vi "CDEx Effect of Controller Type.vi"() -> ()   [LabVIEW 2020]
doc: "This example demonstrate how to calculate the steady-state error for a model with zero, one, or two integrators. This example also demonstrates how to create and simulate a ramp input signal."
uses:
  <vilib>/addons/Control Design/_Model Construction/Data Typedefs.llb/CD Time Info.ctl
  <vilib>/Analysis/1siggen.llb/Ramp Pattern by Samples.vi
  <vilib>/addons/Control Design/_Model Construction/Model Creation.llb/Model Creation SubVI/cd_Create Transfer Function Model.vi
  <vilib>/addons/Control Design/_Utility/Model Viewer.llb/Model Viewer SubVI/cd_Draw Transfer Function Equation (TF).vi
  <vilib>/addons/Control Design/_Model Interconnection/Model Interconnection.llb/Model Interconnection SubVI/cd_Series (TF and TF).vi
  <vilib>/addons/Control Design/_Dynamic Analysis/Dynamic Analysis.llb/Dynamic Analysis subVI/cd_DC Gain (Transfer Function).vi
  <vilib>/addons/Control Design/_Model Interconnection/Model Interconnection.llb/Model Interconnection SubVI/cd_Feedback (TF and TF).vi
  <vilib>/addons/Control Design/_Time Response Analysis/Time Response.llb/Time Response subVI/cd_Linear Simulation (Transfer Function).vi
  <vilib>/addons/Control Design/_Utility/Plots.llb/CD Get IO Time Data.vi
  <vilib>/addons/Control Design/_Time Response Analysis/Time Response.llb/Time Response subVI/cd_Step Response (Transfer Function).vi
  <vilib>/addons/Control Design/_Model Construction/NI_LinSys_Data Typedefs.lvlib
  <vilib>/addons/Control Design/_Dynamic Analysis/NI_CD_Dynamic Analysis.lvlib
  <vilib>/addons/Control Design/_Model Construction/NI_LinSys_Model Creation.lvlib
  <vilib>/addons/Control Design/_Model Interconnection/NI_CD_Model Interconnection.lvlib
  <vilib>/addons/Control Design/_Utility/NI_CD_Model Viewer.lvlib
  <vilib>/addons/Control Design/_Time Response Analysis/NI_CD_Time Response.lvlib
  <vilib>/Analysis/NI_AALBase.lvlib
panel:
  out "Acceleration Error Constant":dbl format="%#.6f"
  out "Steady-state Acceleration Error":dbl=inf format="%#.6f"
  out "Steady-state Velocity Constant (Kv)":dbl=0.27922588002276405 format="%#.6f"
  out "Steady-state Tracking Constant (Kp)":dbl=inf format="%#.6f"
  out "Steady-state Velocity Error":dbl=3.5813299251433084 format="%#.6f"
  out "Steady-state Tracking Error":dbl format="%#.6f"
  in  "Stop":bool
  out "Controller":picture
  in  "Controller Gain":dbl(slide)=0.8376776400682923 scale=0.0001..100.0
  in  "Controller Type":u16(ring)=1 items=["Type 0 - No integrators", "Type 1 - one integrator", "Type 2 - two integrators"]
  out "Plant":picture
  out "Ramp Response":cluster{"time":dbl[], dbl[]}[](graph)
  out "Step Response":cluster{"time":dbl[], dbl[]}[](graph)
  # "Overview: This example demonstrate how to calculate the steady-state error for a model with zero, one, or two integrators.  This example also demonstrates how to create and simulate a ramp input signal.\nInstructions:\n1. Run the VI.\n2. Change the type of Controller and the Controller Gain and verify how this would affect the step and the ramp response. Also, notice that increasing the number of integrators in the plant, it will remove the steady-state error for step or a ramp input signal (u)"
  # "u"
  # "y"
  # "+"
  # "-"
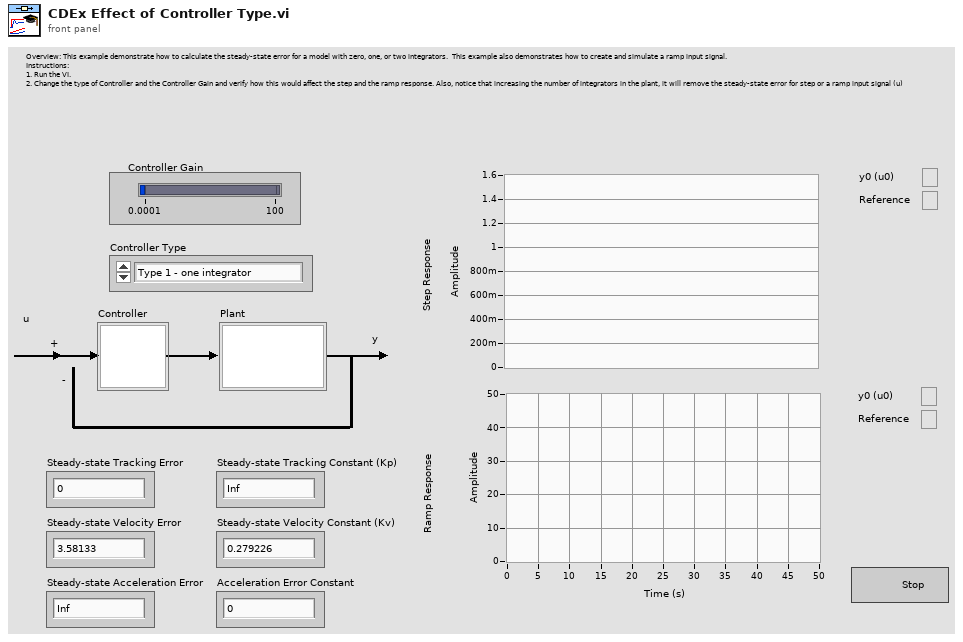
[diagram p1: front panel]
types:
  T1 = typedef "NI_LinSys_Data Typedefs.lvlib/CD Time Info.ctl" = cluster{"t0":dbl, "dt":dbl, "tf":dbl}
  T2 = typedef "NI_LinSys_Model Typedefs.lvlib/CD Transfer Function Model (MIMO).ctl" = cluster{"properties":T3, "transfer function(s)":T4[][]}
  T3 = typedef "NI_LinSys_Model Typedefs.lvlib/CD General Elements.ctl" = cluster{"Model name":string, "Input names":string[], "Output names":string[], "Input Delays":dbl[], "Output Delays":dbl[], "Sampling Time":dbl, "Notes":string}
  T4 = typedef "NI_LinSys_Model Typedefs.lvlib/CD Transfer Function Model (SISO).ctl" = cluster{"Numerator":dbl[], "Denominator":dbl[], "delay":dbl}
  T5 = typedef "NI_LinSys_Data Typedefs.lvlib/CD MIMO Time Response Data.ctl" = cluster{"Time":dbl[], "Outputs Data":dbl[][][], "States Data":dbl[][][], "plot type":T6}
  T6 = typedef "NI_LinSys_Data Typedefs.lvlib/CD Plot Types Enum.ctl" = enum16{"bode-magnitude", "bode-phase", "nichols", "nyquist", "singular values", "step", "impulse", "initial", "simulation", "nyquist with separation"}
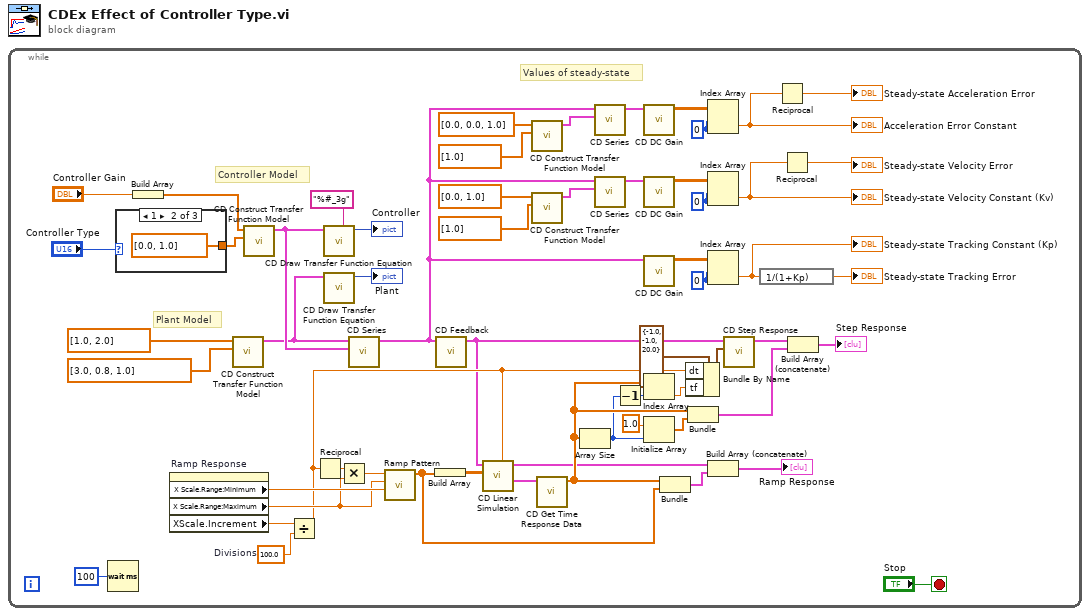
[diagram p0: block diagram]
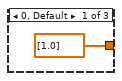
[diagram p2: hidden frame]
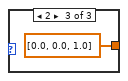
[diagram p3: hidden frame]
diagram:
  n1 = while {
    stop <- "Stop" stop-if-true
    w8 = 0 ("disabled index (col)")
    w20 = 0 ("disabled index (col)")
    w23 = 0 ("disabled index (col)")
    w28 = 100.0  # Divisions
    # "Controller Model"
    # "Plant Model"
    # "Values of steady-state"
    n2 = Wait (ms)(milliseconds to wait=u32 100) -> ()  [unwired: 1 out]
    n3 = case shown="1" "Controller Type" {
      tunnel: [dbl[] [1.0] ("Denominator") dbl[] [0.0, 1.0] ("Denominator") dbl[] [0.0, 0.0, 1.0] ("Denominator")] -> w45
      frame 0, Default {
      }
      frame 1 {
      }
      frame 2 {
      }
    }
    n4 = Build Array("Controller Gain") -> (w39:dbl[])
    n5 = property on="Ramp Response" class="XYGraph (strict)"() -> ("X Scale.Range:Minimum"=w56:dbl, "X Scale.Range:Maximum"=w55:dbl, "XScale.Increment"=w27:dbl)  [unwired: 2 in, 2 out]
    n6 = call-poly <vilib>:"CD Construct Transfer Function Model.vi"("Denominator"=dbl[] [3.0, 0.8, 1.0], "Numerator"=dbl[] [1.0, 2.0]) -> ("Transfer Function Model"=w36:T2)  [unwired: 8 in, 1 out]
    n7 = call-poly <vilib>:"CD Construct Transfer Function Model.vi"("Denominator"=w45, "Numerator"=w39) -> ("Transfer Function Model"=w41:T2)  [unwired: 8 in, 1 out]
    n8 = Divide(x=w27, y=w28) -> (x/y=w26:dbl)
    n9 = Reciprocal(x=w26) -> (1/x=w58:dbl)
    n10 = call-poly <vilib>:"CD Draw Transfer Function Equation.vi"("Format Coefficients"="%#_3g", "Transfer Function Model"=w41) -> ("Equation"=→"Controller":picture)  [unwired: 7 in, 2 out]
    n11 = call-poly <vilib>:"CD Draw Transfer Function Equation.vi"("Transfer Function Model"=w36) -> ("Equation"=→"Plant":picture)  [unwired: 8 in, 2 out]
    n12 = Multiply(x=w58, y=w55) -> (x*y=w57:dbl)
    n13 = call-poly <vilib>:"CD Series.vi"("Model 2"=w41, "Model 1"=w36) -> ("Series Model"=w7:T2)  [unwired: 8 in, 1 out]
    n14 = call-poly <vilib>:"Ramp Pattern.vi"("start"=w56, "end"=w55, "samples"=w57) -> ("Ramp Pattern"=w53:dbl[])  [unwired: 7 in, 1 out]
    n15 = Build Array(w53) -> (w4:dbl[][])
    n16 = call-poly <vilib>:"CD Feedback.vi"("Model 1"=w7) -> ("Closed-Loop Model"=w25:T2)  [unwired: 9 in, 1 out]
    n17 = call-poly <vilib>:"CD Linear Simulation.vi"("Delta t"=w26, "Inputs"=w4, "Transfer Function Model"=w25) -> ("Simulation Data"=w54:T5, "Simulation Graph"=w2:cluster{"time":dbl[], dbl[]}[])  [unwired: 6 in, 1 out]
    n18 = call-poly <vilib>:"CD Construct Transfer Function Model.vi"("Denominator"=dbl[] [1.0], "Numerator"=dbl[] [0.0, 0.0, 1.0]) -> ("Transfer Function Model"=w11:T2)  [unwired: 8 in, 1 out]
    n19 = call-poly <vilib>:"CD Construct Transfer Function Model.vi"("Denominator"=dbl[] [1.0], "Numerator"=dbl[] [0.0, 1.0]) -> ("Transfer Function Model"=w16:T2)  [unwired: 8 in, 1 out]
    n20 = call-poly <vilib>:"CD Get Time Response Data.vi"("Time Response Data"=w54) -> ("Time"=w33:dbl[])  [unwired: 8 in, 2 out]
    n21 = Array Size(array=w33) -> (size(s)=w31:i32)
    n22 = call-poly <vilib>:"CD Series.vi"("Model 2"=w11, "Model 1"=w7) -> ("Series Model"=w12:T2)  [unwired: 8 in, 1 out]
    n23 = call-poly <vilib>:"CD Series.vi"("Model 2"=w16, "Model 1"=w7) -> ("Series Model"=w13:T2)  [unwired: 8 in, 1 out]
    n24 = Decrement(x=w31) -> (x-1=w29:i32)
    n25 = call-poly <vilib>:"CD DC Gain.vi"("Transfer Function Model"=w12) -> ("DC Gain"=w9:dbl[][])  [unwired: 9 in, 1 out]
    n26 = call-poly <vilib>:"CD DC Gain.vi"("Transfer Function Model"=w13) -> ("DC Gain"=w19:dbl[][])  [unwired: 9 in, 1 out]
    n27 = call-poly <vilib>:"CD DC Gain.vi"("Transfer Function Model"=w7) -> ("DC Gain"=w24:dbl[][])  [unwired: 9 in, 1 out]
    n28 = Index Array(array=w33, index=w29) -> (element=w32:dbl)
    n29 = Initialize Array(1.0 ("element"), w31) -> (w49:dbl[])
    n30 = Bundle("Time"=w33, "Ramp Pattern"=w53) -> (w52:cluster{"Time":dbl[], "Ramp Pattern":dbl[]})  [unwired: 1 in]
    n31 = Bundle By Name(cluster=T1 {"t0"=-1.0, "dt"=-1.0, "tf"=20.0} ("Time Info"), "dt"=w26, "tf"=w32) -> (w34:T1)
    n32 = Bundle("Time"=w33, w49) -> (w48:cluster{"Time":dbl[], dbl[]})  [unwired: 1 in]
    n33 = Index Array(array=w9, index (row)=w8, index (col)=w8) -> (element=w6:dbl)
    "Acceleration Error Constant" <- w6
    n34 = Index Array(array=w19, index (row)=w20, index (col)=w20) -> (element=w15:dbl)
    "Steady-state Velocity Constant (Kv)" <- w15
    n35 = Index Array(array=w24, index (row)=w23, index (col)=w23) -> (element=w21:dbl)
    "Steady-state Tracking Constant (Kp)" <- w21
    n36 = Build Array (concatenate)(w2, w52) -> (→"Ramp Response":cluster{"Time":dbl[], "Ramp Pattern":dbl[]}[])
    n37 = call-poly <vilib>:"CD Step Response.vi"("Time Range"=w34, "Transfer Function Model"=w25) -> ("Step Response Graph"=w51:cluster{"time":dbl[], dbl[]}[])  [unwired: 7 in, 2 out]
    n38 = expression code="1/(1+Kp)"(w21) -> (→"Steady-state Tracking Error":dbl)
    n39 = Reciprocal(x=w6) -> (1/x=→"Steady-state Acceleration Error":dbl)
    n40 = Reciprocal(x=w15) -> (1/x=→"Steady-state Velocity Error":dbl)
    n41 = Build Array (concatenate)(w51, w48) -> (→"Step Response":cluster{"Time":dbl[], dbl[]}[])
  }
